vi "mqttCmdCreate.vi"(8 "error in (no error)":errorcluster) -> (0 "error out":errorcluster, 3 "mqttCmdConnect out":refnum<class "mqttCmdConnect.lvclass">)   [LabVIEW 2020, in "mqttCmdConnect.lvclass"]
uses:
  mqttCmdConnect.lvclass
  C:/Projects/Libraries/Gore SM 2020/mqtt-LabVIEW/src/class/mqtt/mqttCmd/mqttCmd.lvclass
  mqtt.lvclass
  mqttTypedef/mqttQOSlevel.ctl
  mqttTypedef/mqttMessageType.ctl
  mqtt.lvclass/mqtt.ctl
  mqttCmd.lvclass/mqttCmd.ctl
  Read keepAlive(sec).vi
  Read clientID.vi
  Read connFlags.vi
  Properties/Read User Info.vi
  Read Will Info.vi
  Properties/Write Datagram.vi
  mqttCmd.lvclass
panel:
  in  "mqtt instance":refnum<class "mqtt.lvclass">
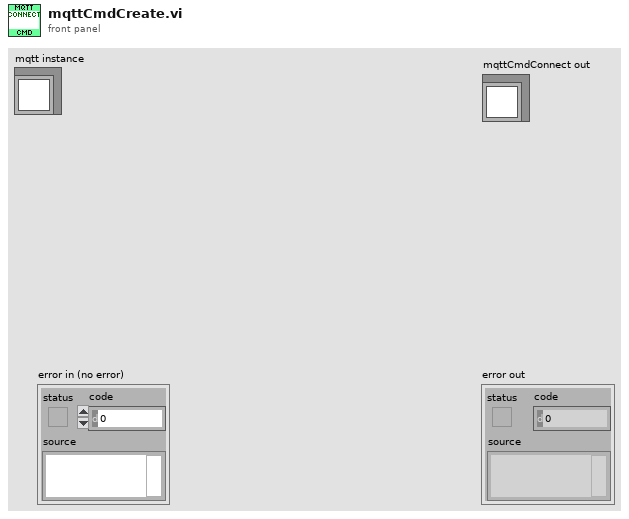
[diagram p1: front panel]
types:
  T1 = typedef "mqttMessageType.ctl" = enum32{"Reserved", "CONNECT", "CONNACK", "PUBLISH", "PUBACK", "PUBREC", "PUBREL", "PUBCOMP", "SUBSCRIBE", "SUBACK", "UNSUBSCRIBE", "UNSUBACK", "PINGREQ", "PINGRESP", "DISCONNECT", "Reserved2"}
  T2 = typedef "mqttQOSlevel.ctl" = enum8{"At most once", "At least once", "Exactly once", "Reserved"}
  T3 = typedef "mqttConnectionFlags.ctl" = cluster{"reserved":bool, "clean session":bool, "will flag":bool, "willQOS":enum8{"At most once", "At least once", "Exactly once", "Reserved"}, "will retain":bool, "password":bool, "user name":bool}
  T4 = typedef "mqttWillInformation.ctl" = cluster{"User Name":string, "Password":string}
  T5 = typedef "mqttUserInformation.ctl" = cluster{"Will message":string, "Will Topic":string}
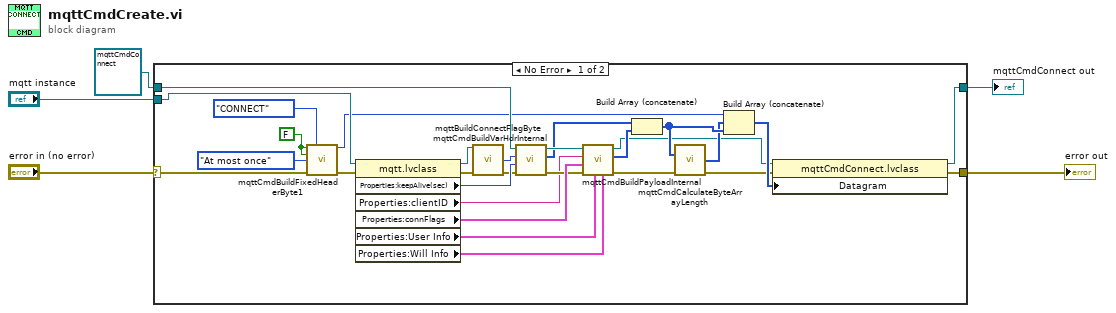
[diagram p0: block diagram]
diagram:
  n1 = case shown="No Error" "error in (no error)" {
    selector: "error in (no error)" -> [w13 w36]
    tunnel: [w19 w36] -> w4
    tunnel: [w32 w35] -> w1
    tunnel: "mqtt instance" -> [w31 _]
    tunnel: refnum<class "mqttCmdConnect.lvclass"> refnum ("mqttCmdConnect out") -> [w26 w35]
    frame No Error {
      w16 = FALSE
      n2 = call "mqttCmdBuildFixedHeaderByte1.vi"("retain(F)"=w16, "MessageType"=mqttMessageType."CONNECT", "duplicate(F)"=w16, "QoS (At most once)"=mqttQOSlevel."At most once", "error in (no error)"=w13) -> ("byte1"=w14:u8, "error out"=w12:errorcluster)  [unwired: 9 in]
      n3 = property class="mqtt.lvclass"(reference=w31, error in=w12) -> (reference out=w9:refnum<class "mqtt.lvclass">, error out=w8:errorcluster, "Properties:keepAlive(sec)"=w10:u16, "Properties:clientID"=w11:string, "Properties:connFlags"=w30:T3, "Properties:User Info"=w29:T4, "Properties:Will Info"=w28:T5)
      n4 = call "mqttBuildConnectFlagByte.vi"("mqtt in"=w9, "error in (no error)"=w8) -> ("connFlagByte out"=w6:u8, "error out"=w7:errorcluster)  [unwired: 11 in, 1 out]
      n5 = call "mqttCmdBuildVarHdrInternal.vi"("error in (no error)"=w7, "keepAlive(sec)"=w10, "connFlagByte"=w6, "mqttCmdConnect in"=w26) -> ("error out"=w24:errorcluster, "varHeader"=w23:u8[], "mqttCmdConnect out"=w25:refnum<class "mqttCmdConnect.lvclass">)  [unwired: 5 in]
      n6 = call "mqttCmdBuildPayloadInternal.vi"("Will Info"=w28, "User Info"=w29, "error in (no error)"=w24, "connFlags"=w30, "ClientID"=w11, "mqttCmdConnect in"=w25) -> ("error out"=w21:errorcluster, "payload"=w27:u8[], "mqttCmdConnect out"=w18:refnum<class "mqttCmdConnect.lvclass">)  [unwired: 3 in]
      n7 = Build Array (concatenate)(w23, w27) -> (w34:u8[])
      n8 = call "mqttCmdCalculateByteArrayLength.vi"("byteArry in"=w34, "error in (no error)"=w21) -> ("length out"=w33:u8[], "error out"=w20:errorcluster)  [unwired: 12 in]
      n9 = Build Array (concatenate)(w14, w33, w34) -> (w22:u8[])
      n10 = property class="mqttCmdConnect.lvclass"(reference=w18, error in=w20, "Datagram"=w22) -> (reference out=w32:refnum<class "mqttCmdConnect.lvclass">, error out=w19:errorcluster)
    }
    frame Error {
    }
  }
  "error out" <- w4
  "mqttCmdConnect out" <- w1
